vi "Get Bucket Logging.vi"(8 "error in (no error)":errorcluster, 11 "Bucket in":refnum<class "Bucket.lvclass">) -> (0 "error out":errorcluster, 2 "Logging Status":T1, 3 "Bucket out":refnum<class "Bucket.lvclass">)   [LabVIEW 2015, in "NI_AWS_S3.lvlib" / "Bucket.lvclass"]
uses:
  Bucket.lvclass
  Logging Status.ctl
  Logging Grantee-Permission Pair.ctl
  Logging Permission.ctl
  Core/HTTP Request/Region handling.ctl
  Core/HTTP Request/Request Options.ctl
  Core/HTTP Request/Name Value Pair.ctl
  Core/HTTP Request/URL formatting.ctl
  Bucket.lvclass/Bucket.ctl
  Read Name.vi
  Core/HTTP Request/HTTP Request.lvclass
  XML Parsing/NI_XML Parsing.lvlib
  NI_AWS_S3.lvlib
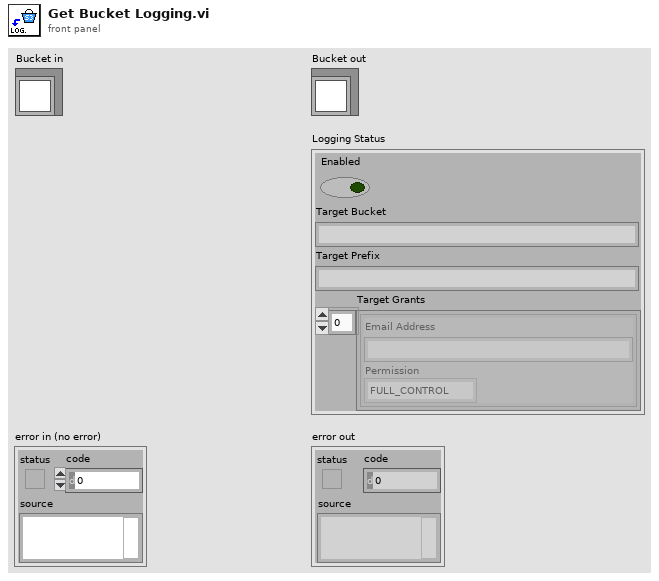
[diagram p1: front panel]
types:
  T1 = typedef "NI_AWS_S3.lvlib/Logging Status.ctl" = cluster{"Enabled":bool, "Target Bucket":string, "Target Prefix":string, "Target Grants":T2[]}
  T2 = typedef "NI_AWS_S3.lvlib/Logging Grantee-Permission Pair.ctl" = cluster{"Email Address":string, "Permission":T3}
  T3 = typedef "NI_AWS_S3.lvlib/Logging Permission.ctl" = enum16{"FULL_CONTROL", "READ", "WRITE"}
  T4 = typedef "NI_AWS_Core.lvlib/HTTP Request.lvclass/Name Value Pair.ctl" = cluster{"name":string, "value":string}
  T5 = typedef "NI_AWS_Core.lvlib/HTTP Request.lvclass/Request Options.ctl" = cluster{"request headers":T4[], "request parameters":T4[], "request body":string, "region handling":T6, "URL formatting":T7}
  T6 = typedef "NI_AWS_Core.lvlib/HTTP Request.lvclass/Region handling.ctl" = enum16{"use region everywhere", "use region (authentication only)", "use region (URL only)", "ignore region everwhere"}
  T7 = typedef "NI_AWS_Core.lvlib/HTTP Request.lvclass/URL formatting.ctl" = enum16{"region-", "region."}
  T8 = typedef "NI_AWS_Core.lvlib/HTTP Request.lvclass/Response.ctl" = cluster{"Headers":string, "Body":string}
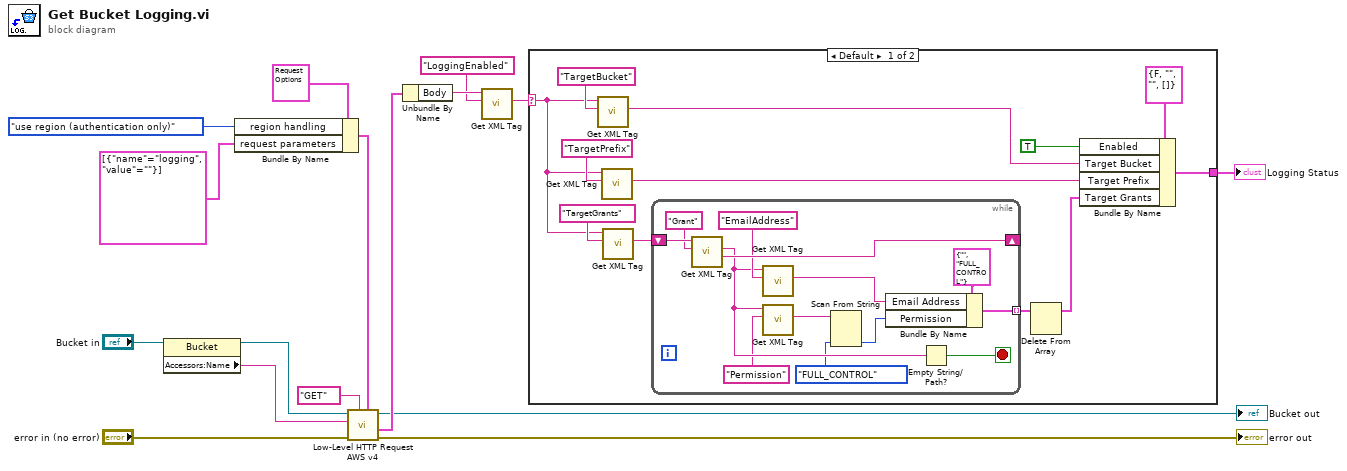
[diagram p0: block diagram]
diagram:
  n1 = property class="Bucket"(reference="Bucket in") -> (reference out=w5:refnum<class "Bucket.lvclass">, "Accessors:Name"=w16:string)  [unwired: 1 in, 1 out]
  n2 = Bundle By Name(cluster=T5 {"request headers"=[], "request parameters"=[], "request body"="", "region handling"=enum."use region everywhere", "URL formatting"=enum."region."} ("Request Options"), "region handling"=Region_handling."use region (authentication only)", "request parameters"=T4[] [{"name"="logging", "value"=""}]) -> (w6:T5)
  n3 = call "Low-Level HTTP Request AWS v4.vi"("Request Options"=w6, "HTTP-Verb"="GET", "error in (no error)"="error in (no error)", "URL Prefix"=w16, "AWS Core in"=w5) -> ("error out"=→"error out":errorcluster, "Response"=w8:T8, "AWS Core out"=→"Bucket out":refnum<class "Bucket.lvclass">)  [unwired: 3 in, 1 out]
  n4 = Unbundle By Name(w8) -> ("Body"=w9:string)
  n5 = call "Get XML Tag.vi"("Tag name"="LoggingEnabled", "XML String in"=w9) -> ("Tag value"=w2:string)  [unwired: 5 in, 4 out]
  n6 = case shown="Default" w2 {
    selector: w2 -> [w20 _]
    tunnel: [w27 _] -> w1
    frame Default {
      n7 = call "Get XML Tag.vi"("Tag name"="TargetBucket", "XML String in"=w20) -> ("Tag value"=w24:string)  [unwired: 5 in, 4 out]
      n8 = call "Get XML Tag.vi"("Tag name"="TargetPrefix", "XML String in"=w20) -> ("Tag value"=w22:string)  [unwired: 5 in, 4 out]
      n9 = call "Get XML Tag.vi"("Tag name"="TargetGrants", "XML String in"=w20) -> ("Tag value"=w19:string)  [unwired: 5 in, 4 out]
      n10 = while {
        shift-right: [w37] -> _
        shift-left: w19 -> [w39]
        tunnel: [w40] -> w18 mode=indexing
        stop <- w36 stop-if-true
        n11 = call "Get XML Tag.vi"("Tag name"="Grant", "XML String in"=w39) -> ("Remaining string"=w37:string, "Tag value"=w33:string)  [unwired: 5 in, 3 out]
        n12 = call "Get XML Tag.vi"("Tag name"="EmailAddress", "XML String in"=w33) -> ("Tag value"=w34:string)  [unwired: 5 in, 4 out]
        n13 = call "Get XML Tag.vi"("Tag name"="Permission", "XML String in"=w33) -> ("Tag value"=w31:string)  [unwired: 5 in, 4 out]
        n14 = Scan From String(input string=w31, default 1=Logging_Permission."FULL_CONTROL" ("Permission")) -> (output 1=w30:T3)  [unwired: 3 in, 3 out]
        n15 = Bundle By Name(cluster=T2 {"Email Address"="", "Permission"=enum."FULL_CONTROL"} ("Logging Grantee-Permission Pair"), "Email Address"=w34, "Permission"=w30) -> (w40:T2)
        n16 = Empty String/Path?(string/path=w33) -> (empty?=w36:bool)
      }
      n17 = Delete From Array(array=w18) -> (array with subset deleted=w17:T2[])  [unwired: 2 in, 1 out]
      n18 = Bundle By Name(cluster=T1 {"Enabled"=FALSE, "Target Bucket"="", "Target Prefix"="", "Target Grants"=[]} ("Logging Status"), "Enabled"=TRUE, "Target Bucket"=w24, "Target Prefix"=w22, "Target Grants"=w17) -> (w27:T1)
    }
    frame "" {
    }
  }
  "Logging Status" <- w1
